vi "Configure Digital Output Port.vi"(8 "error in (no error)":errorcluster, 9 "Enable Output Port State (False)":bool, 10 "Output Port Number (0)":i32, 11 "VISA resource name":refnum<visa-resource-name>) -> (0 "error out":errorcluster, 3 "VISA resource name out":refnum<visa-resource-name>)   [LabVIEW 2017, in "HH PLI Series.lvlib"]
doc: "Configures digital output ports of the Analog I/O Port."
uses:
  HH PLI Series.lvlib
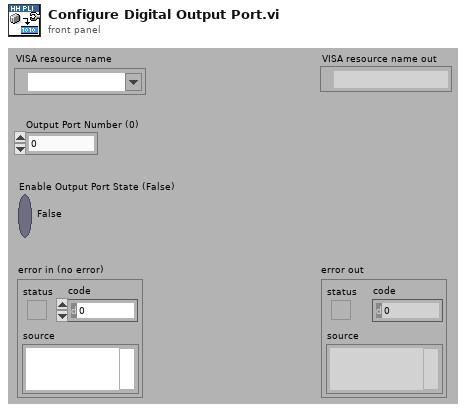
[diagram p1: front panel]
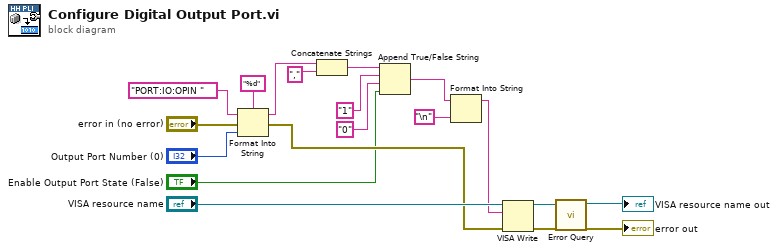
[diagram p0: block diagram]
diagram:
  n1 = Format Into String(format string="%d", initial string="PORT:IO:OPIN " ("command"), error in="error in (no error)", "Output Port Number (0)") -> (resulting string=w15:string, error out=w16:errorcluster)
  n2 = Concatenate Strings(w15, "," ("command")) -> (w9:string)
  n3 = Append True/False String(1:"Enable Output Port State (False)", 2:"0" ("false string"), 3:"1" ("true string"), 4:w9) -> (0:w2:string)
  n4 = Format Into String(initial string=w2, "\n") -> (resulting string=w1:string)  [unwired: 2 in, 1 out]
  n5 = VISA Write(VISA resource name="VISA resource name", write buffer=w1, error in (no error)=w16) -> (VISA resource name out=w6:refnum<visa-resource-name>, error out=w7:errorcluster)  [unwired: 1 out]
  n6 = call "Error Query.vi"("error in (no error)"=w7, "VISA resource name"=w6) -> ("error out"=→"error out":errorcluster, "VISA resource name out"=→"VISA resource name out":refnum<visa-resource-name>)  [unwired: 6 in, 2 out]
